vi "FRCts20_WebMethods_Cluster2HTML.vi"(8 "error in (no error)":errorcluster, 11 "Cluster":variant) -> (0 "error out":errorcluster, 3 "HTML":string)   [LabVIEW 2014]
uses:
  FRCts20_WebMethods.lvlib
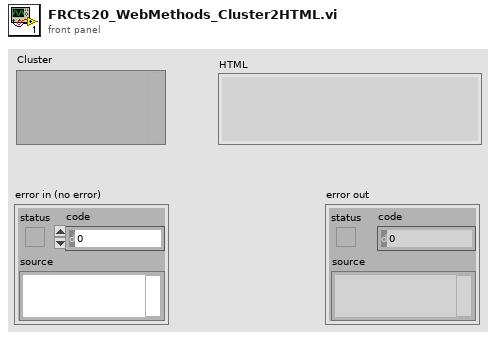
[diagram p1: front panel]
types:
  T1 = enum16{"(default)", "monospaced", "italic", "bold", "underlined", "strike-through", "big", "small", "superscript", "subscript"}
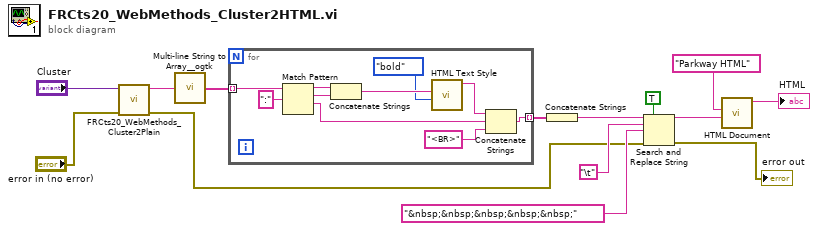
[diagram p0: block diagram]
diagram:
  n1 = call "FRCts20_WebMethods_Cluster2Plain.vi"("error in (no error)"="error in (no error)", "Cluster"="Cluster") -> ("error out"=w2:errorcluster, "plain text"=w9:string)  [unwired: 8 in]
  n2 = call <userlib>:"Multi-line String to Array__ogtk.vi"("string"=w9) -> ("lines"=w8:string[])
  n3 = for {
    tunnel: w8 -> [w24] mode=indexing
    tunnel: [w16] -> w7 mode=indexing
    n4 = Match Pattern(string=w24, regular expression=":") -> (before substring=w22:string, match substring=w21:string, after substring=w17:string)  [unwired: 1 in, 1 out]
    n5 = Concatenate Strings(w22, w21) -> (w20:string)
    n6 = call <vilib>:"HTML Text Style.vi"("style (default)"=T1."bold", "text"=w20) -> ("HTML out"=w18:string)  [unwired: 9 in]
    n7 = Concatenate Strings(w18, w17, "<BR>") -> (w16:string)
  }
  n8 = Concatenate Strings(w7) -> (w3:string)
  n9 = Search and Replace String(replace all?=TRUE ("replace all? (F)"), input string=w3, search string="\t", replace string="&nbsp;&nbsp;&nbsp;&nbsp;&nbsp;", error in=w2) -> (result string=w4:string, error out=→"error out":errorcluster)  [unwired: 3 in, 2 out]
  n10 = call <vilib>:"HTML Document.vi"("document body"=w4, "document title"="Parkway HTML") -> ("HTML Document"=→"HTML":string)  [unwired: 9 in]
